vi "reverse_indices.vi"(2 "indices":i32[](array[numeric])) -> (7 "reverse indices":i32[](array[numeric]))   [LabVIEW 2015]
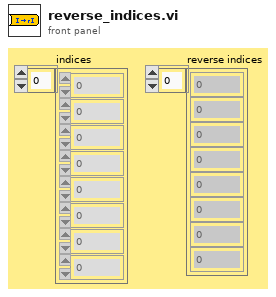
[diagram p1: front panel]
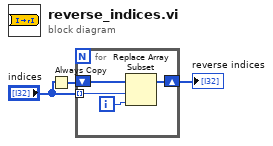
[diagram p0: block diagram]
diagram:
  n1 = Always Copy(1:"indices") -> (0:w2:i32[])
  n2 = for {
    tunnel: "indices" -> [w7] mode=indexing
    shift-right: [w5] -> w1
    shift-left: w2 -> [w6]
    i -> [w4]
    n3 = Replace Array Subset(array=w6, new element=w4, index=w7) -> (w5:i32[])
  }
  "reverse indices" <- w1
